vi "Sub Read Img Json Data.vi"(8 "error in":errorcluster, 10 "File Data":T1, 11 "PNG Path":path) -> (0 "error out":errorcluster, 2 "Image Path":path, 3 "Json Data":T2)   [LabVIEW 2018, in "Main Panel.lvlib" / "Main Panel.lvclass"]
uses:
  Main Panel.lvclass
  Image Json Parser/Img Json Data.ctl
  Image Json Parser/Img Json Frames.ctl
  Image Json Parser/Img Json Meta.ctl
  Frame Analizer/Bmp File Data.ctl
  Image Json Parser/Image Json Parser.lvclass
  Frame Analizer/Data Parser.lvclass
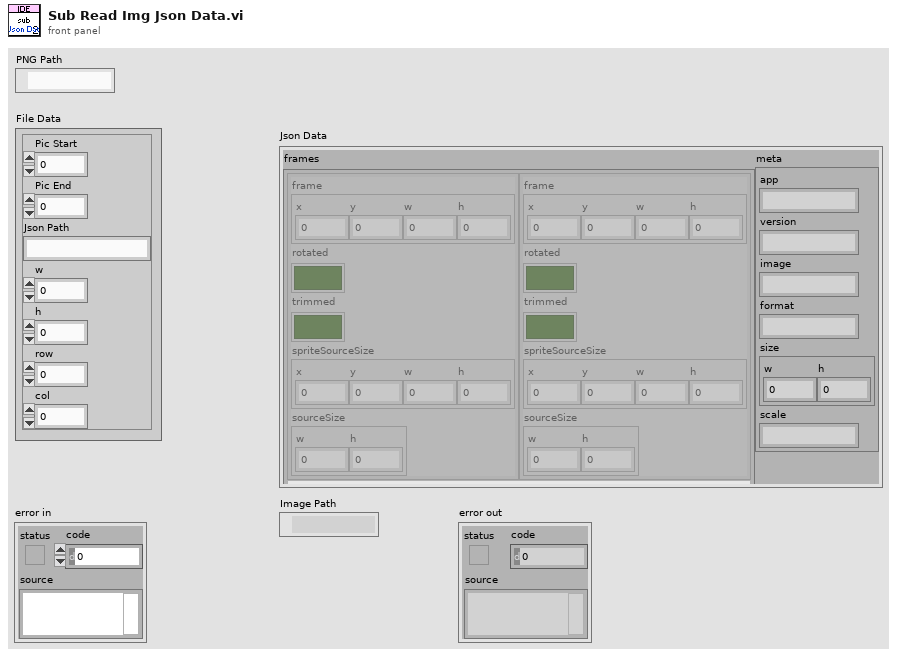
[diagram p1: front panel]
types:
  T1 = typedef "Data Parser.lvclass/Bmp File Data.ctl" = cluster{"Pic Start":i32, "Pic End":i32, "Json Path":string, "w":i32, "h":i32, "row":i32, "col":i32}
  T2 = typedef "Image Json Parser.lvclass/Img Json Data.ctl" = cluster{"frames":T3[], "meta":T4}
  T3 = typedef "Image Json Parser.lvclass/Img Json Frames.ctl" = cluster{"frame":cluster{"x":i32, "y":i32, "w":i32, "h":i32}, "rotated":bool, "trimmed":bool, "spriteSourceSize":cluster{"x":i32, "y":i32, "w":i32, "h":i32}, "sourceSize":cluster{"w":i32, "h":i32}}
  T4 = typedef "Image Json Parser.lvclass/Img Json Meta.ctl" = cluster{"app":string, "version":string, "image":string, "format":string, "size":cluster{"w":i32, "h":i32}, "scale":string}
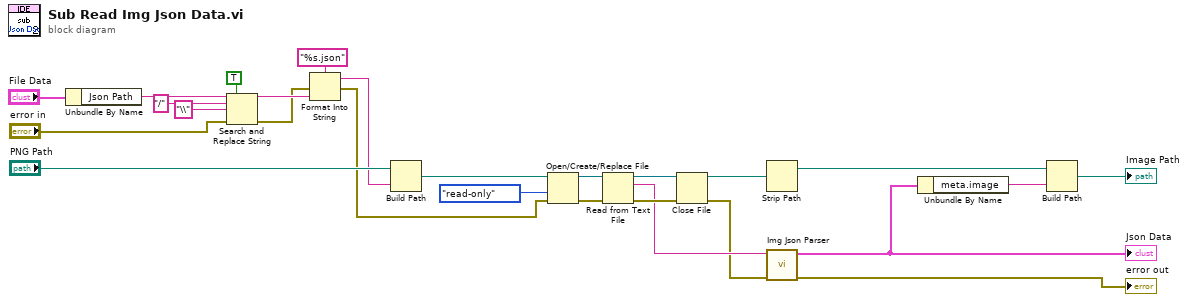
[diagram p0: block diagram]
diagram:
  n1 = Unbundle By Name("File Data") -> ("Json Path"=w14:string)
  n2 = Search and Replace String(replace all?=TRUE ("replace all? (F)"), input string=w14, search string="/", replace string="\\" ("replace string (\"\")"), error in="error in") -> (result string=w13:string, error out=w12:errorcluster)  [unwired: 3 in, 2 out]
  n3 = Format Into String(format string="%s.json", error in=w12, w13) -> (resulting string=w15:string, error out=w17:errorcluster)  [unwired: 1 in]
  n4 = Build Path(base path="PNG Path", name or relative path=w15) -> (appended path=w19:path)
  n5 = Open/Create/Replace File(file path (use dialog)=w19, error in=w17, access (0:read/write)=enum16{"read/write", "read-only", "write-only"}."read-only") -> (refnum out=w24:refnum<file>, error out=w23:errorcluster)  [unwired: 3 in, 1 out]
  n6 = Read from Text File(file (use dialog)=w24, error in=w23) -> (refnum out=w22:refnum<file>, text=w16:string, error out=w21:errorcluster)  [unwired: 2 in, 1 out]
  n7 = Close File(refnum=w22, error in=w21) -> (path=w5:path, error out=w8:errorcluster)
  n8 = Strip Path(path=w5) -> (stripped path=w4:path)  [unwired: 1 out]
  n9 = call "Img Json Parser.vi"("error in (no error)"=w8, "Json string"=w16) -> ("error out"=→"error out":errorcluster, "Json data"=w3:T2)  [unwired: 7 in, 1 out]
  "Json Data" <- w3
  n10 = Unbundle By Name(w3) -> ("meta.image"=w2:string)
  n11 = Build Path(base path=w4, name or relative path=w2) -> (appended path=→"Image Path":path)
